vi "lab2_new_p1.vi"() -> ()   [LabVIEW 2021]
panel:
  out "Numeric":dbl
  in  "N":dbl
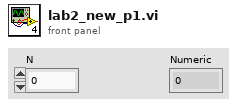
[diagram p1: front panel]
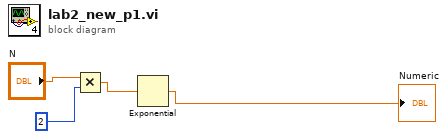
[diagram p0: block diagram]
diagram:
  n1 = Multiply(x="N", y=2) -> (x*y=w2:dbl)
  n2 = Exponential(1:w2) -> (0:→"Numeric":dbl)
